vi "Single Z Ramp Experiment.vi"(0 "Initial Phase Offset":dbl, 1 "Experimental Queue":T1) -> ()   [LabVIEW 2013]
uses:
  Runtime/Runtime Queue.ctl
  Runtime/Experimental Configuration.ctl
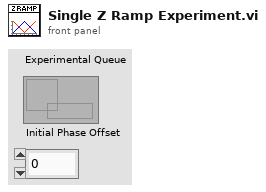
[diagram p1: front panel]
types:
  T1 = typedef "Runtime Queue.ctl" = refnum<queue>
  T2 = typedef "Experimental Configuration.ctl" = cluster{"Output Waveforms":waveform(dbl)[], "Output Channels":string, "Input Channels":string, "DAQ Data Notifier Name":string}
  T3 = cluster{"Z Position Data":dbl[], "Force Data":dbl[]}
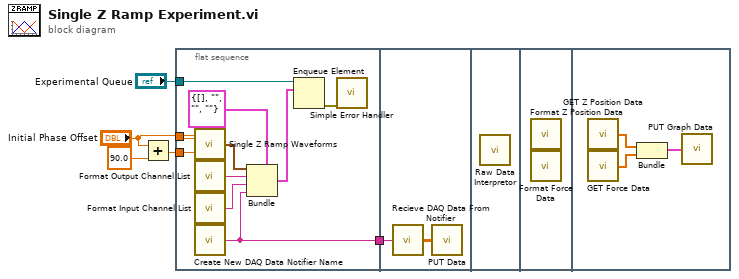
[diagram p0: block diagram]
diagram:
  n1 = Add(x="Initial Phase Offset", y=90.0) -> (x+y=w3:dbl)
  n2 = flat-sequence {
    tunnel: "Experimental Queue" -> [w15]
    tunnel: w3 -> [w8]
    tunnel: "Initial Phase Offset" -> [w7]
    tunnel: [w6] -> w1
    tunnel: w1 -> [w16]
    frame #0 {
      n3 = call "Single Z Ramp Waveforms.vi"("Second Phase Offset"=w8, "Initial Phase Offset"=w7) -> ("Output Waveforms"=w11:waveform(dbl)[])
      n4 = call "Format Output Channel List.vi"() -> ("Output Channels"=w13:string)
      n5 = call "Format Input Channel List.vi"() -> ("Input Channels"=w12:string)
      n6 = call "Create New DAQ Data Notifier Name.vi"() -> ("Notifier Name"=w6:string)
      n7 = Bundle(cluster=T2 {"Output Waveforms"=[], "Output Channels"="", "Input Channels"="", "DAQ Data Notifier Name"=""} ("Experimental Configuration"), "Output Waveforms"=w11, "Output Channels"=w13, "Input Channels"=w12, "DAQ Data Notifier Name"=w6) -> (w10:T2)
      n8 = Enqueue Element(queue=w15, element=w10) -> (error out=w14:errorcluster)  [unwired: 2 in, 2 out]
      n9 = call <vilib>:"Simple Error Handler.vi"("error in (no error)"=w14) -> ()  [unwired: 4 in, 5 out]
    }
    frame #1 {
      n10 = call "Recieve DAQ Data From Notifier.vi"("Notifier Name"=w16) -> ("Experimental Data"=w17:dbl[][])
      n11 = call "PUT Data.vi"("Data"=w17) -> ()
    }
    frame #2 {
      n12 = call "Raw Data Interpretor.vi"() -> ()  [unwired: 1 in]
    }
    frame #3 {
      n13 = call "Format Z Position Data.vi"() -> ()  [unwired: 1 in]
      n14 = call "Format Force Data.vi"() -> ()  [unwired: 1 in]
    }
    frame #4 {
      n15 = call "GET Z Position Data.vi"() -> ("Z Position Data"=w18:dbl[])
      n16 = call "GET Force Data.vi"() -> ("Force Data"=w19:dbl[])
      n17 = Bundle("Z Position Data"=w18, "Force Data"=w19) -> (w20:T3)  [unwired: 1 in]
      n18 = call "PUT Graph Data.vi"("Graph Data"=w20) -> ()
    }
  }
